vi "correct_zero_crossing_times.vi"(9 "p->n idõk":dbl[](array[numeric]), 10 "n->p idõk":dbl[](array[numeric]), 11 "csúcs idõk":dbl[](array[numeric])) -> (2 "korrigált p->n idõk":dbl[](array[numeric]), 3 "korrigált n->p idõk":dbl[](array[numeric]))   [LabVIEW 2017]
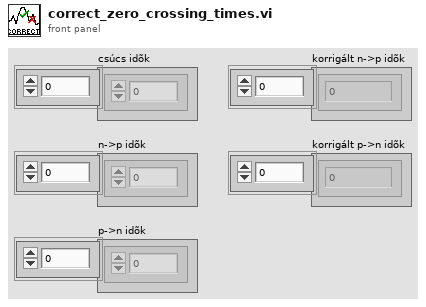
[diagram p1: front panel]
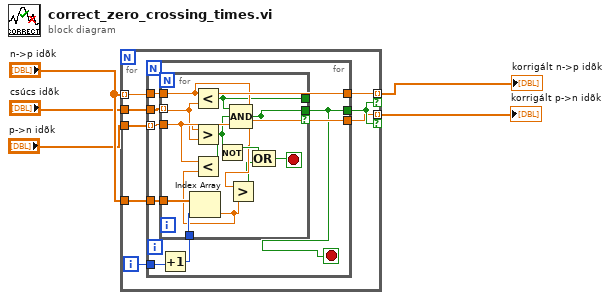
[diagram p0: block diagram]
diagram:
  n1 = for {
    tunnel: "n->p idõk" -> [w10] mode=indexing
    tunnel: "p->n idõk" -> [w12]
    tunnel: "csúcs idõk" -> [w11]
    tunnel: [w9] -> w1 mode=indexing if=w13
    tunnel: [w8] -> w2 mode=indexing if=w13
    tunnel: "n->p idõk" -> [w7]
    i -> [w6]
    n2 = for {
      tunnel: [w17] -> w13
      tunnel: w12 -> [w18] mode=indexing
      tunnel: w11 -> [w20]
      tunnel: w10 -> [w19]
      tunnel: [w19] -> w9
      tunnel: [w18] -> w8
      tunnel: w7 -> [w16]
      tunnel: w6 -> [w14]
      stop <- w17 stop-if-true
      n3 = Increment(x=w14) -> (x+1=w15:i32)
      n4 = for {
        tunnel: [w26] -> w17 if=w26
        tunnel: w18 -> [w22]
        tunnel: w20 -> [w33] mode=indexing
        tunnel: w19 -> [w28]
        tunnel: [w25] -> _
        tunnel: w15 -> [w29]
        tunnel: w16 -> [w30]
        stop <- w31 stop-if-true
        n5 = Index Array(array=w30, index=w29) -> (element=w21:dbl)
        n6 = Less?(x=w28, y=w33) -> (x < y?=w25:bool)
        n7 = Greater?(x=w22, y=w33) -> (0:w24:bool)
        n8 = Less?(x=w22, y=w21) -> (x < y?=w23:bool)
        n9 = Not(x=w24) -> (.not. x?=w32:bool)
        n10 = Greater?(x=w28, y=w21) -> (0:w27:bool)
        n11 = Compound Arithmetic op=AND(w25, w24, w23) -> (w26:bool)
        n12 = Compound Arithmetic op=OR(w32, w27) -> (w31:bool)
      }
    }
  }
  "korrigált p->n idõk" <- w2
  "korrigált n->p idõk" <- w1
